vi "Is Child Path.vi"(10 "File":path, 11 "Base Folder":path) -> (1 "is Child Path":bool, 2 "relative path from Base to File":path)   [LabVIEW 2020, in "Save for Previous Version.lvlib"]
uses:
  Save for Previous Version.lvlib
  <userlib>/_OpenG.lib/file/file.llb/Valid Path - Traditional__ogtk.vi
  <userlib>/_OpenG.lib/file/file.llb/Compare Two Paths - Scalar__ogtk.vi
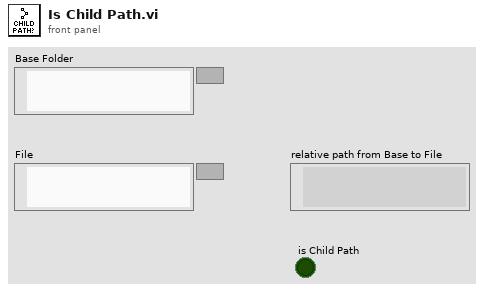
[diagram p1: front panel]
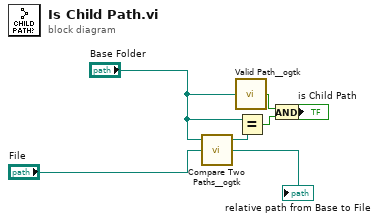
[diagram p0: block diagram]
diagram:
  n1 = call-poly <userlib>:"Compare Two Paths__ogtk.vi"("path2"="File", "path1"="Base Folder") -> ("relative path from 1 to 2"=→"relative path from Base to File":path, "common path"=w2:path)  [unwired: 1 in, 1 out]
  n2 = call-poly <userlib>:"Valid Path__ogtk.vi"("path"="Base Folder") -> ("valid"=w3:bool)
  n3 = Equal?(x="Base Folder", y=w2) -> (x = y?=w4:bool)
  n4 = And(x=w3, y=w4) -> (x .and. y?=→"is Child Path":bool)
